vi "Read Results.vi"(10 "Results Indexes":T3, 11 "result allocation in":T2) -> (2 "Cluster":T1, 3 "data table out":T2)   [LabVIEW 2015, in "Sequencer Module tests.lvlib"]
uses:
  Sequencer Module tests.lvlib
  Results Indexes.ctl
  <vilib>/NI/Tag Bus/table/data table.ctl
  Results.ctl
  <vilib>/NI/Tag Bus/table/data polymorphs/read one/read Boolean.vi
  <vilib>/NI/Tag Bus/table/data polymorphs/read one/read I32.vi
  <vilib>/NI/Tag Bus/table/data table.lvlib
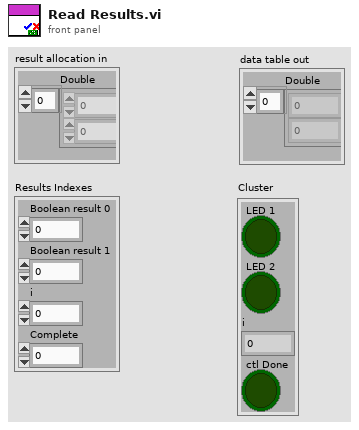
[diagram p1: front panel]
types:
  T1 = typedef "Sequencer Module tests.lvlib/Results.ctl" = cluster{"LED 1":bool, "LED 2":bool, "i":i32, "ctl Done":bool}
  T2 = typedef "tag bus.lvlib/data table.lvlib/data table.ctl" = cluster{"Double":dbl[], "Single":sgl[], "I64":i64[], "I32":i32[], "I16":i16[], "I8":i8[], "U64":u64[], "U32":u32[], "U16":u16[], "U8":u8[], "Boolean":bool[], "String":string[], "Array of Double":cluster{"DBL Array":dbl[]}[], "Array of Single":cluster{"SGL Array":sgl[]}[], "Array of I64":cluster{"I64 Array":i64[]}[], "Array of I32":cluster{"I32 Array":i32[]}[], "Array of I16":cluster{"I16 Array":i16[]}[], "Array of I8":cluster{"I8 Array":i8[]}[], "Array of U64":cluster{"U64 Array":u64[]}[], "Array of U32":cluster{"U32 Array":u32[]}[], "Array of U16":cluster{"U16 Array":u16[]}[], "Array of U8":cluster{"U8 Array":u8[]}[], "Array of Boolean":cluster{"Boolean Array":bool[]}[], "Array of String":cluster{"String Array":string[]}[]}
  T3 = typedef "Sequencer Module tests.lvlib/Results Indexes.ctl" = cluster{"Boolean result 0":i32, "Boolean result 1":i32, "i":i32, "Complete":i32}
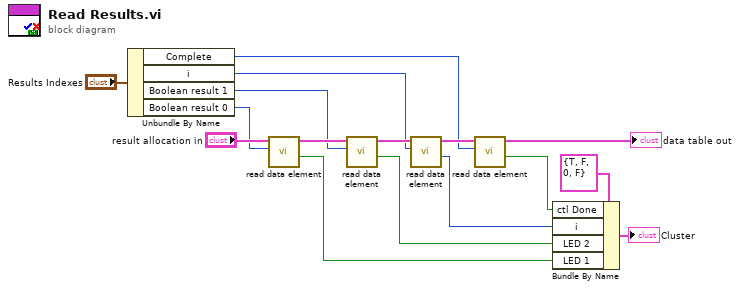
[diagram p0: block diagram]
diagram:
  n1 = Unbundle By Name("Results Indexes") -> ("Complete"=w7:i32, "i"=w6:i32, "Boolean result 1"=w5:i32, "Boolean result 0"=w4:i32)
  n2 = call-poly <vilib>:"read data element.vi"("index"=w4, "data table in"="result allocation in") -> ("value"=w3:bool, "data table out"=w13:T2)  [unwired: 8 in]
  n3 = call-poly <vilib>:"read data element.vi"("index"=w5, "data table in"=w13) -> ("value"=w2:bool, "data table out"=w15:T2)  [unwired: 8 in]
  n4 = call-poly <vilib>:"read data element.vi"("index"=w6, "data table in"=w15) -> ("value"=w1:i32, "data table out"=w14:T2)  [unwired: 8 in]
  n5 = call-poly <vilib>:"read data element.vi"("index"=w7, "data table in"=w14) -> ("value"=w9:bool, "data table out"=→"data table out":T2)  [unwired: 8 in]
  n6 = Bundle By Name(cluster=T1 {"LED 1"=TRUE, "LED 2"=FALSE, "i"=0, "ctl Done"=FALSE} ("Cluster"), "ctl Done"=w9, "i"=w1, "LED 2"=w2, "LED 1"=w3) -> (→"Cluster":T1)
